vi "ClosestPeak_Window.vi"(7 "Range":T1={"X_Min"=0.3, "X_Max"=0.3, "Y_Min"=0.3, "Y-Max"=0.3}, 8 "Window Width (point)":i32=80, 9 "The Data":dbl[](array[numeric]) format="%.2f", 10 "X-axis":dbl[](array[numeric]) format="%.2f", 11 "Searching center":dbl format="%.2f") -> (0 "Data Subset":dbl[](array[numeric]) format="%.2f", 1 "X-Axis Subset":dbl[](array[numeric]) format="%.2f", 3 "Closest peak position":dbl format="%.2f", 4 "starting point":dbl format="%.2f", 5 "scale":dbl format="%.2f")   [LabVIEW 2019]
doc: "Truncate the data around a peak. Normalize X-Axis so I can use the spline VI, and you can retrive the original X-Axis with *scale+StartingPoint."
uses:
  <vilib>/Analysis/NI_AALPro.lvlib
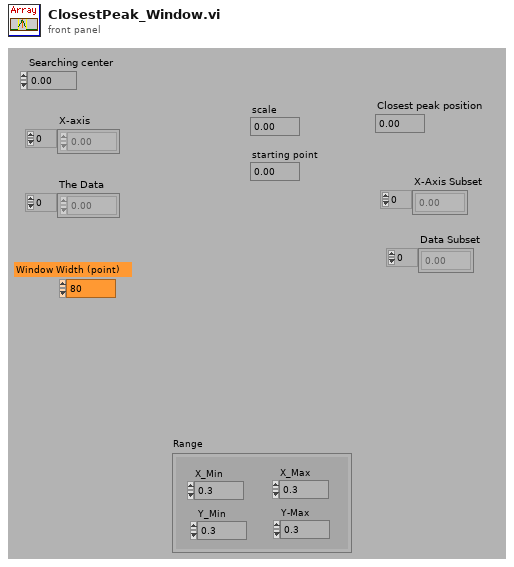
[diagram p1: front panel]
types:
  T1 = cluster{"X_Min":dbl, "X_Max":dbl, "Y_Min":dbl, "Y-Max":dbl}
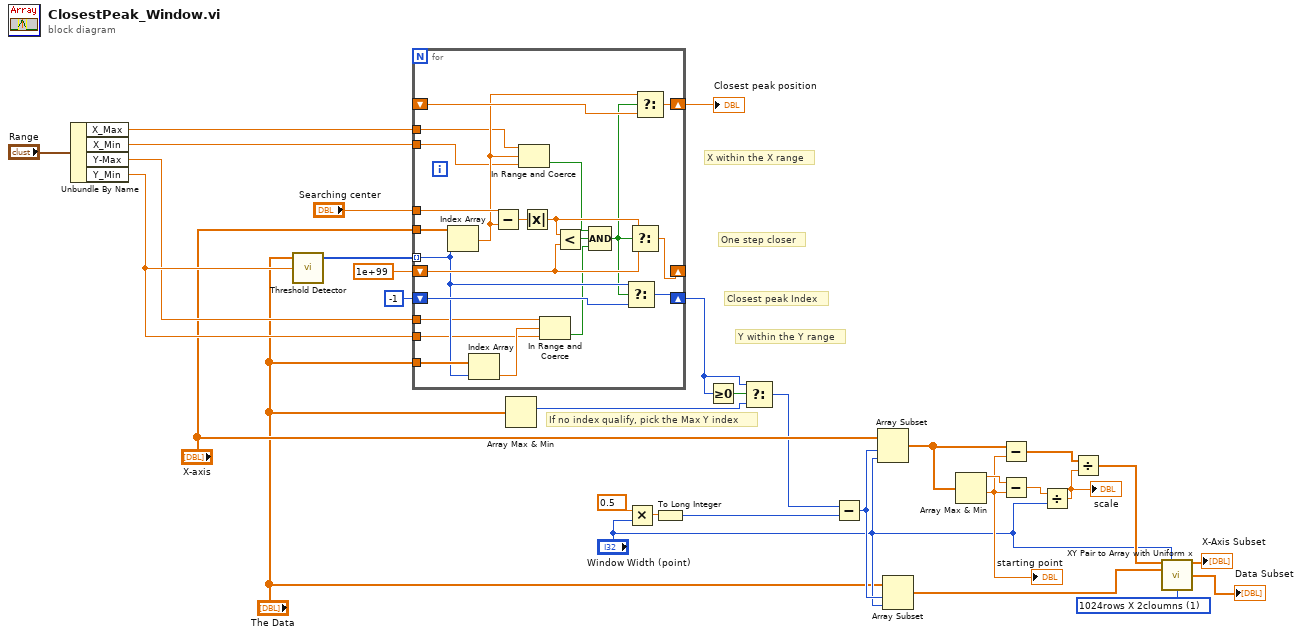
[diagram p0: block diagram]
diagram:
  w13 = u8 1 items=["No Change", "1024rows X 2cloumns", "1024X2 Fixed Endpoints"] ("Data Format")
  # "If no index qualify, pick the Max Y index"
  # "One step closer"
  # "Y within the Y range"
  # "X within the X range"
  # "Closest peak Index"
  n1 = Unbundle By Name("Range") -> ("X_Max"=w8:dbl, "X_Min"=w9:dbl, "Y-Max"=w10:dbl, "Y_Min"=w11:dbl)
  n2 = call <vilib>:"Threshold Detector.vi"("threshold"=w11, "X"="The Data") -> ("Indices"=w29:i32[])  [unwired: 1 in, 2 out]
  n3 = for {
    tunnel: w29 -> [w43] mode=indexing
    tunnel: "X-axis" -> [w54]
    tunnel: "Searching center" -> [w53]
    shift-right: [w49] -> _
    shift-left: 1e+99 ("x") -> [w50]
    shift-right: [w48] -> w32
    shift-left: _ -> [w47]
    shift-right: [w46] -> w3
    shift-left: -1 -> [w45]
    tunnel: "The Data" -> [w44]
    tunnel: w11 -> [w41]
    tunnel: w10 -> [w40]
    tunnel: w9 -> [w38]
    tunnel: w8 -> [w37]
    n4 = Index Array(array=w54, index=w43) -> (element=w39:dbl)
    n5 = Index Array(array=w44, index=w43) -> (element=w42:dbl)
    n6 = Subtract(x=w53, y=w39) -> (x-y=w52:dbl)
    n7 = In Range and Coerce(upper limit=w37, x=w39, lower limit=w38) -> (In Range?=w36:bool)  [unwired: 1 out]
    n8 = Absolute Value(x=w52) -> (abs(x)=w51:dbl)
    n9 = In Range and Coerce(upper limit=w40, x=w42, lower limit=w41) -> (In Range?=w33:bool)  [unwired: 1 out]
    n10 = Less?(x=w51, y=w50) -> (x < y?=w34:bool)
    n11 = Compound Arithmetic op=AND(w36, w34, w33) -> (w35:bool)
    n12 = Select(t=w43, s=w35, f=w45) -> (s? t:f=w46:i32)
    n13 = Select(t=w51, s=w35, f=w50) -> (s? t:f=w49:dbl)
    n14 = Select(t=w39, s=w35, f=w47) -> (s? t:f=w48:dbl)
  }
  "Closest peak position" <- w32
  n15 = Array Max & Min(array="The Data") -> (max index (indices)=w2:i32)  [unwired: 3 out]
  n16 = Multiply(x=sgl 0.5 ("y"), y="Window Width (point)") -> (x*y=w28:sgl)
  n17 = To Long Integer(number=w28) -> (32bit integer=w27:i32)
  n18 = Greater Or Equal To 0?(x=w3) -> (x >= 0?=w4:bool)
  n19 = Select(t=w3, s=w4, f=w2) -> (s? t:f=w1:i32)
  n20 = Subtract(x=w1, y=w27) -> (x-y=w25:i32)
  n21 = Array Subset(array="X-axis", index=w25, length="Window Width (point)") -> (w21:dbl[])
  n22 = Array Subset(array="The Data", index=w25, length="Window Width (point)") -> (w17:dbl[])
  n23 = Array Max & Min(array=w21) -> (max value=w24:dbl, min value=w22:dbl)  [unwired: 2 out]
  "starting point" <- w22
  n24 = Subtract(x=w21, y=w22) -> (x-y=w20:dbl[])
  n25 = Subtract(x=w24, y=w22) -> (x-y=w23:dbl)
  n26 = Divide(x=w23, y="Window Width (point)") -> (x/y=w19:dbl)
  "scale" <- w19
  n27 = Divide(x=w20, y=w19) -> (x/y=w18:dbl[])
  n28 = call "XY Pair to Array with Uniform x.vi"("x"=w18, "#Points"="Window Width (point)", "y"=w17, "Data Format"=w13) -> ("X output"=→"X-Axis Subset":dbl[], "Y output"=→"Data Subset":dbl[])  [unwired: 10 in]
